vi "Create Param Filter.vi"(7 "Param Size":enum16{"Scalar", "1d", "2d"}(ring), 8 "error in":errorcluster, 9 "Model Section":refnum<k24>) -> (0 "error out":errorcluster, 1 "Model Section dup":refnum<k24>, 4 "Filter":refnum<k24>)   [LabVIEW 2011]
uses:
  NationalInstruments.VeriStand.SystemStorage
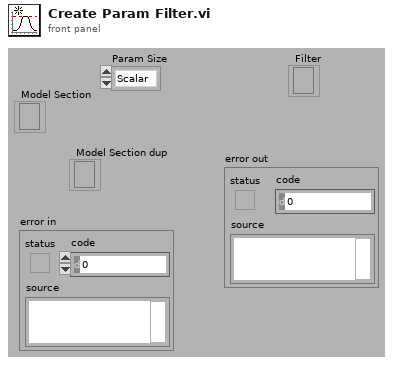
[diagram p1: front panel]
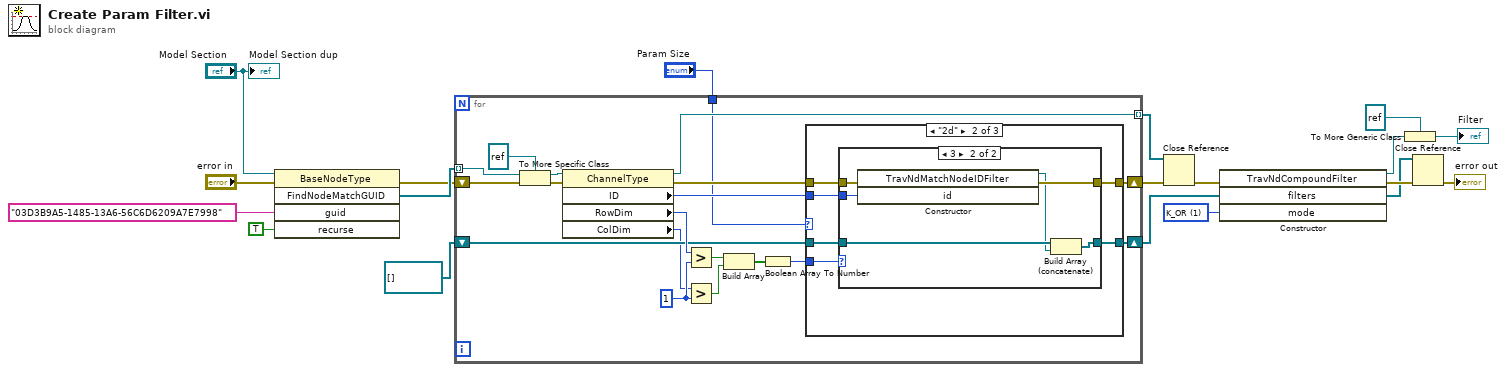
[diagram p0: block diagram]
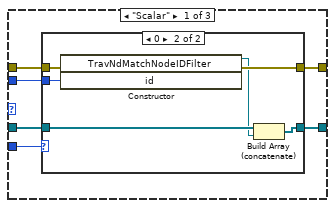
[diagram p2: hidden frame]
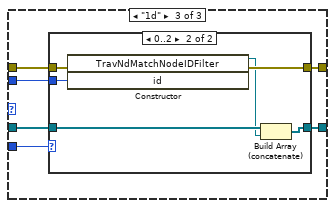
[diagram p5: hidden frame]
diagram:
  w19 = 1 items=["K_AND", "K_OR"] ("mode")
  n1 = invoke class="BaseNodeType" method="FindNodeMatchGUID"(reference="Model Section", error in="error in", "guid"="03D3B9A5-1485-13A6-56C6D6209A7E7998", "recurse"=TRUE) -> (error out=w11:errorcluster, "FindNodeMatchGUID"=w12:refnum<k24>[])  [unwired: 1 in, 3 out]
  n2 = for {
    tunnel: w12 -> [w37] mode=indexing
    shift-right: [w24] -> w13
    shift-left: w11 -> [w38]
    tunnel: [w33] -> w14 mode=indexing
    shift-right: [w26] -> w18
    shift-left: refnum<k24>[] [] -> [w27]
    tunnel: "Param Size" -> [w22]
    w31 = 1 ("y")
    n3 = To More Specific Class(target class=refnum<k24> refnum, reference=w37, error in=w38) -> (specific class reference=w35:refnum<k24>, error out=w34:errorcluster)
    n4 = property class="ChannelType"(reference=w35, error in=w34) -> (reference out=w33:refnum<k24>, error out=w25:errorcluster, "ID"=w23:u64, "RowDim"=w32:i32, "ColDim"=w20:i32)
    n5 = Greater?(x=w32, y=w31) -> (0:w30:bool)
    n6 = Greater?(x=w20, y=w31) -> (0:w29:bool)
    n7 = Build Array(w30, w29) -> (w28:bool[])
    n8 = Boolean Array To Number(Boolean array=w28) -> (number=w21:u32)
    n9 = case shown="\"2d\"" w22 {
      tunnel: w21 -> [w40 w54 w72]
      tunnel: w27 -> [w41 w55 w71]
      tunnel: [w39 w53 w70] -> w26
      tunnel: w25 -> [w43 w57 w69]
      tunnel: [w44 w58 w68] -> w24
      tunnel: w23 -> [w42 w56 w67]
      frame "Scalar" {
        n10 = case shown="0" w40 {
          tunnel: w41 -> [w46 w52]
          tunnel: [w46 w51] -> w39
          tunnel: w43 -> [w45 w50]
          tunnel: [w45 w49] -> w44
          tunnel: w42 -> [_ w48]
          frame Default {
          }
          frame 0 {
            n11 = constructor class="TravNdMatchNodeIDFilter"(error in=w50, "id"=w48) -> (reference out=w47:refnum<k24>, error out=w49:errorcluster)  [unwired: 2 in, 2 out]
            n12 = Build Array (concatenate)(w52, w47) -> (w51:refnum<k24>[])
          }
        }
      }
      frame "2d" {
        n13 = case shown="3" w54 {
          tunnel: w55 -> [w60 w66]
          tunnel: [w60 w65] -> w53
          tunnel: w57 -> [w59 w64]
          tunnel: [w59 w63] -> w58
          tunnel: w56 -> [_ w62]
          frame Default {
          }
          frame 3 {
            n14 = constructor class="TravNdMatchNodeIDFilter"(error in=w64, "id"=w62) -> (reference out=w61:refnum<k24>, error out=w63:errorcluster)  [unwired: 2 in, 2 out]
            n15 = Build Array (concatenate)(w66, w61) -> (w65:refnum<k24>[])
          }
        }
      }
      frame "1d" {
        n16 = case shown="0..2" w72 {
          tunnel: w71 -> [w74 w80]
          tunnel: [w74 w79] -> w70
          tunnel: w69 -> [w73 w78]
          tunnel: [w73 w77] -> w68
          tunnel: w67 -> [_ w76]
          frame Default {
          }
          frame 0..2 {
            n17 = constructor class="TravNdMatchNodeIDFilter"(error in=w78, "id"=w76) -> (reference out=w75:refnum<k24>, error out=w77:errorcluster)  [unwired: 2 in, 2 out]
            n18 = Build Array (concatenate)(w80, w75) -> (w79:refnum<k24>[])
          }
        }
      }
    }
  }
  n19 = Close Reference(reference=w14, error in (no error)=w13) -> (error out=w17:errorcluster)
  n20 = constructor class="TravNdCompoundFilter"(error in=w17, "filters"=w18, "mode"=w19) -> (reference out=w6:refnum<k24>, error out=w3:errorcluster, "filters"=w2:refnum<k24>[])  [unwired: 2 in, 2 out]
  n21 = To More Generic Class(target class=refnum<k24> refnum, reference=w6) -> (generic class reference=→"Filter":refnum<k24>)
  n22 = Close Reference(reference=w2, error in (no error)=w3) -> (error out=→"error out":errorcluster)
  "Model Section dup" <- "Model Section"
